vi "Add SLSC Module To Chassis.vi"(7 "Name":string, 8 "error in (no error)":errorcluster, 9 "Slot Number":u32=1, 10 "SLSC Custom Device XML":path, 11 "SLSC Chassis":u64) -> (0 "error out":errorcluster, 2 "SLSC Module":u64, 3 "SLSC Chassis out":u64)   [LabVIEW 2020, in "VeriStand SLSC Scripting.lvlib"]
uses:
  VeriStand SLSC Scripting.lvlib
  Controls/SLSC Custom Device Information.ctl
  Controls/Custom Device Information.ctl
  Controls/Dependent File Information.ctl
  <vilib>/NI VeriStand/Custom Device API/Custom Device Supported Target.ctl
  <vilib>/NI VeriStand/Custom Device API/Custom Device API.lvlib
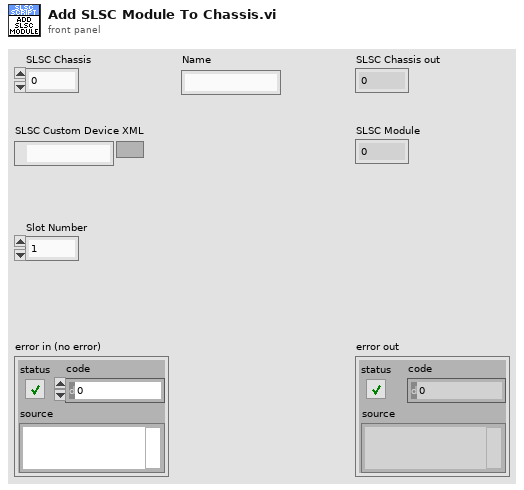
[diagram p1: front panel]
types:
  T1 = typedef "VeriStand SLSC Scripting.lvlib/SLSC Custom Device Information.ctl" = cluster{"Custom Device Information":T2, "Slot #":i32}
  T2 = typedef "VeriStand SLSC Scripting.lvlib/Custom Device Information.ctl" = cluster{"Execution Mode":i32, "Version":string, "Driver VIs":T3[], "Dependencies":T3[], "Main Page GUID":string, "Add Menu":string}
  T3 = typedef "VeriStand SLSC Scripting.lvlib/Dependent File Information.ctl" = cluster{"Path":string, "Type":i32, "Supported Target":T4, "RT System Destination":string, "Version":string, "MD5":string}
  T4 = typedef "Custom Device API.lvlib/Custom Device Supported Target.ctl" = enum16{"All", "PharLap", "VxWorks", "Windows", "Linux_32_ARM", "Linux_x64", "PharLap & Windows", "PharLap & VxWorks", "VxWorks & Windows"}
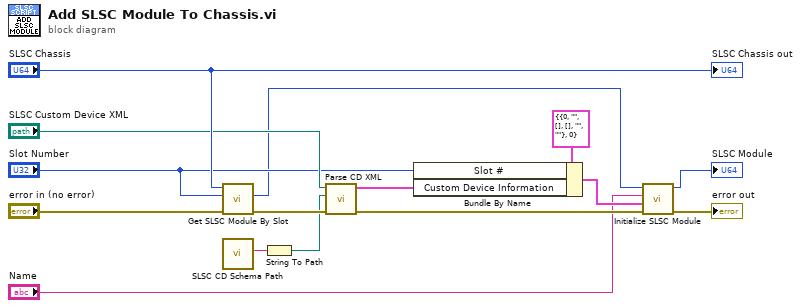
[diagram p0: block diagram]
diagram:
  n1 = call "Get SLSC Module By Slot.vi"("error in (no error)"="error in (no error)", "Slot"="Slot Number", "SLSC Chassis"="SLSC Chassis") -> ("error out"=w12:errorcluster, "SLSC Module"=w4:u64)  [unwired: 6 in, 1 out]
  n2 = call "SLSC CD Schema Path.vi"() -> ("SLSC CD Schema Path"=w13:string)  [unwired: 11 in]
  n3 = String To Path(string=w13) -> (path=w10:path)
  n4 = call "Parse CD XML.vi"("error in (no error)"=w12, "Custom Device XML Schema"=w10, "Custom Device XML"="SLSC Custom Device XML") -> ("error out"=w7:errorcluster, "Custom Device Information"=w6:T2)  [unwired: 7 in]
  n5 = Bundle By Name(cluster=T1 {"Custom Device Information"={"Execution Mode"=0, "Version"="", "Driver VIs"=[], "Dependencies"=[], "Main Page GUID"="", "Add Menu"=""}, "Slot #"=0} ("SLSCCDInfo"), "Slot #"="Slot Number", "Custom Device Information"=w6) -> (w8:T1)
  n6 = call "Initialize SLSC Module.vi"("error in (no error)"=w7, "SLSC Custom Device Information"=w8, "Name"="Name", "SLSC Module"=w4) -> ("error out"=→"error out":errorcluster, "SLSC Module out"=→"SLSC Module":u64)  [unwired: 6 in]
  "SLSC Chassis out" <- "SLSC Chassis"
